vi "Memory.Pointer.Errors.Write Pointer Size.vi"(9 "offset":i32, 10 "error in":errorcluster, 11 "pointer in":refnum<class "Memory.Pointer.lvclass">) -> (1 "new offset":i32, 2 "error out":errorcluster, 3 "pointer out":refnum<class "Memory.Pointer.lvclass">)   [LabVIEW 2016, in "Memory Manager.lvlib" / "Memory.Pointer.lvclass"]
uses:
  Memory.Pointer.lvclass
  Memory.Pointer.lvclass/Memory.Pointer.ctl
  Submodules/Static Error Handling/Source/Library/VIs/Static Error Handling.Source Buffer.Write.Numeric.Scalar.Base10 (U64).vi
  Submodules/Static Error Handling/Source/Library/Static Error Handling.lvlib
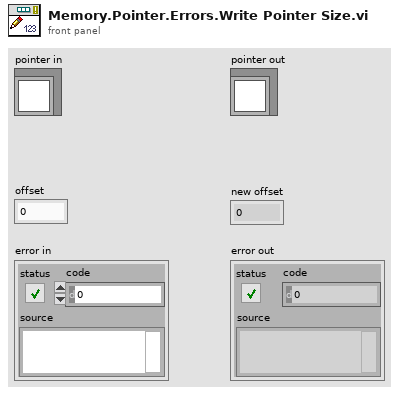
[diagram p1: front panel]
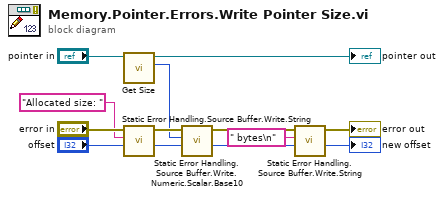
[diagram p0: block diagram]
diagram:
  n1 = call "Get Size.vi"("Pointer in"="pointer in") -> ("size"=w6:u64, "Pointer out"=→"pointer out":refnum<class "Memory.Pointer.lvclass">)  [unwired: 8 in, 1 out]
  n2 = call "Static Error Handling.Source Buffer.Write.String.vi"("offset"="offset", "string"="Allocated size: ", "error in"="error in") -> ("new offset"=w12:i32, "error out"=w13:errorcluster)  [unwired: 7 in]
  n3 = call-poly "Static Error Handling.Source Buffer.Write.Numeric.Scalar.Base10.vi"("offset"=w12, "value"=w6, "error in"=w13) -> ("new offset"=w4:i32, "error out"=w5:errorcluster)  [unwired: 7 in]
  n4 = call "Static Error Handling.Source Buffer.Write.String.vi"("offset"=w4, "string"=" bytes\n", "error in"=w5) -> ("new offset"=→"new offset":i32, "error out"=→"error out":errorcluster)  [unwired: 7 in]
